vi "Move SBlock Up.vi"(8 "error in (no error)":errorcluster, 10 "index":i32, 11 "Sequence of SBlocks in":refnum<class "Sequence of SBlocks.lvclass">) -> (0 "error out":errorcluster, 2 "New Index":i32, 3 "Sequence of SBlocks out":refnum<class "Sequence of SBlocks.lvclass">)   [LabVIEW 2020, in "Run Utilities.lvlib" / "Sequence of SBlocks.lvclass"]
uses:
  Sequence of SBlocks.lvclass
  Sequence of SBlocks.lvclass/Sequence of SBlocks.ctl
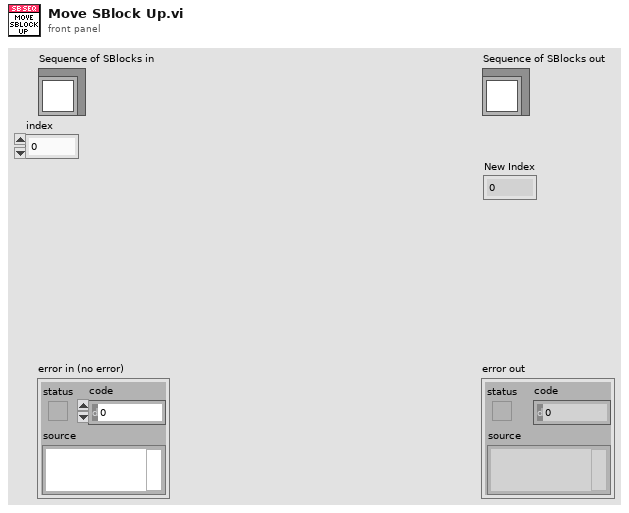
[diagram p1: front panel]
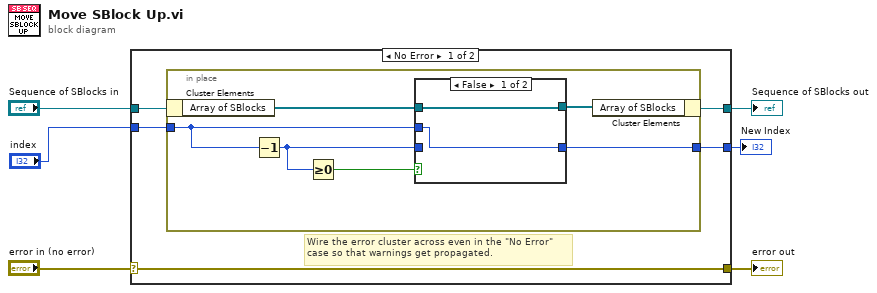
[diagram p0: block diagram]
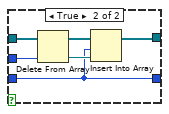
[diagram p2: hidden frame]
diagram:
  n1 = case shown="No Error" "error in (no error)" {
    selector: "error in (no error)" -> [w11 w28]
    tunnel: [w11 w28] -> w5
    tunnel: [w9 w27] -> w3
    tunnel: "Sequence of SBlocks in" -> [w10 w27]
    tunnel: "index" -> [w8 w26]
    tunnel: [w7 w26] -> w1
    frame No Error {
      # "Wire the error cluster across even in the \"No Error\"\ncase so that warnings get propagated."
      n2 = in-place {
        in-place-border: w8 -> [w16]
        in-place-border: [w12] -> w7
        n3 = in-place-cluster #1(w10) -> ("Array of SBlocks"=w17:refnum<class "Schedule Block.lvclass">[])
        n4 = Decrement(x=w16) -> (x-1=w14:i32)
        n5 = Greater Or Equal To 0?(x=w14) -> (x >= 0?=w13:bool)
        n6 = case shown="False" w13 {
          tunnel: w17 -> [w19 w25]
          tunnel: w16 -> [w18 w22]
          tunnel: [w19 w21] -> w15
          tunnel: w14 -> [_ w20]
          tunnel: [w18 w20] -> w12
          frame False {
          }
          frame True {
            n7 = Delete From Array(array=w25, index=w22) -> (deleted portion=w23:refnum<class "Schedule Block.lvclass">, array with subset deleted=w24:refnum<class "Schedule Block.lvclass">[])  [unwired: 1 in]
            n8 = Insert Into Array(array=w24, index=w20, new element=w23) -> (w21:refnum<class "Schedule Block.lvclass">[])
          }
        }
        n9 = in-place-cluster #1("Array of SBlocks"=w15) -> (w9:refnum<class "Sequence of SBlocks.lvclass">)
      }
    }
    frame Error {
    }
  }
  "error out" <- w5
  "Sequence of SBlocks out" <- w3
  "New Index" <- w1
